vi "FindFacesAndSendToServer.vi"(8 "error in":errorcluster, 11 "Image In":T1) -> (0 "error out":errorcluster)   [LabVIEW 2019]
uses:
  <vilib>/vision/Image Controls.llb/IMAQ Image.ctl
panel:
  in  "File Path":path
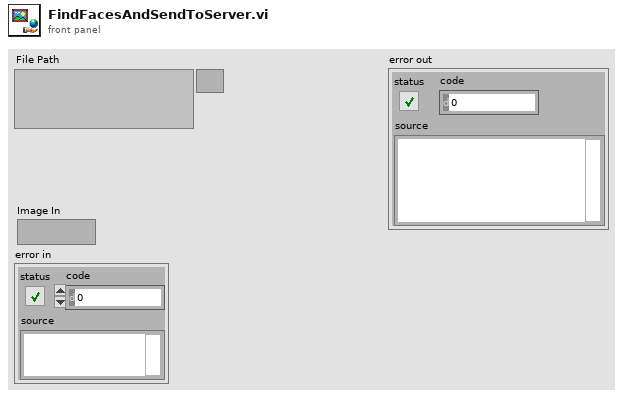
[diagram p1: front panel]
types:
  T1 = typedef "IMAQ Image.ctl" = refnum<image>
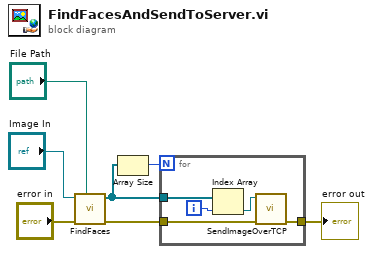
[diagram p0: block diagram]
diagram:
  n1 = call "FindFaces.vi"("File Path"="File Path", "error in"="error in", "Image In"="Image In") -> ("error out"=w2:errorcluster, "Array"=w6:T1[])  [unwired: 7 in]
  n2 = Array Size(array=w6) -> (size(s)=w3:i32)
  n3 = for {
    N: w3 -> [_]
    tunnel: w6 -> [w12]
    tunnel: [w10] -> w1
    tunnel: w2 -> [w8]
    i -> [w9]
    n4 = Index Array(array=w12, index=w9) -> (element=w11:T1)
    n5 = call "SendImageOverTCP.vi"("error in (no error)"=w8, "Image"=w11) -> ("error out"=w10:errorcluster)  [unwired: 9 in]
  }
  "error out" <- w1
